vi "AIT 664 - Parse DB.vi"(0 "Path in":path=path "C:/Users/benh/Desktop/Simple Device Export.xml", 11 "error in (no error)":errorcluster) -> (4 "664 Device":T1, 15 "error out":errorcluster)   [LabVIEW 2015, in "AIT 664 Custom Device.lvlib"]
doc: "Read in xml configuration file and merge with params file if it exists"
uses:
  AIT 664 Custom Device.lvlib
  Controls/664 - XML Device Description.ctl
  Controls/664 - XML End System Description.ctl
  Controls/664 - XML Output VL.ctl
  Controls/664 - XML Tx Message Port.ctl
  Controls/664 - Sampling Type.ctl
  Controls/664 -Param.ctl
  Controls/664 - XML Input VL.ctl
  Controls/664 - XML Rx Message Port.ctl
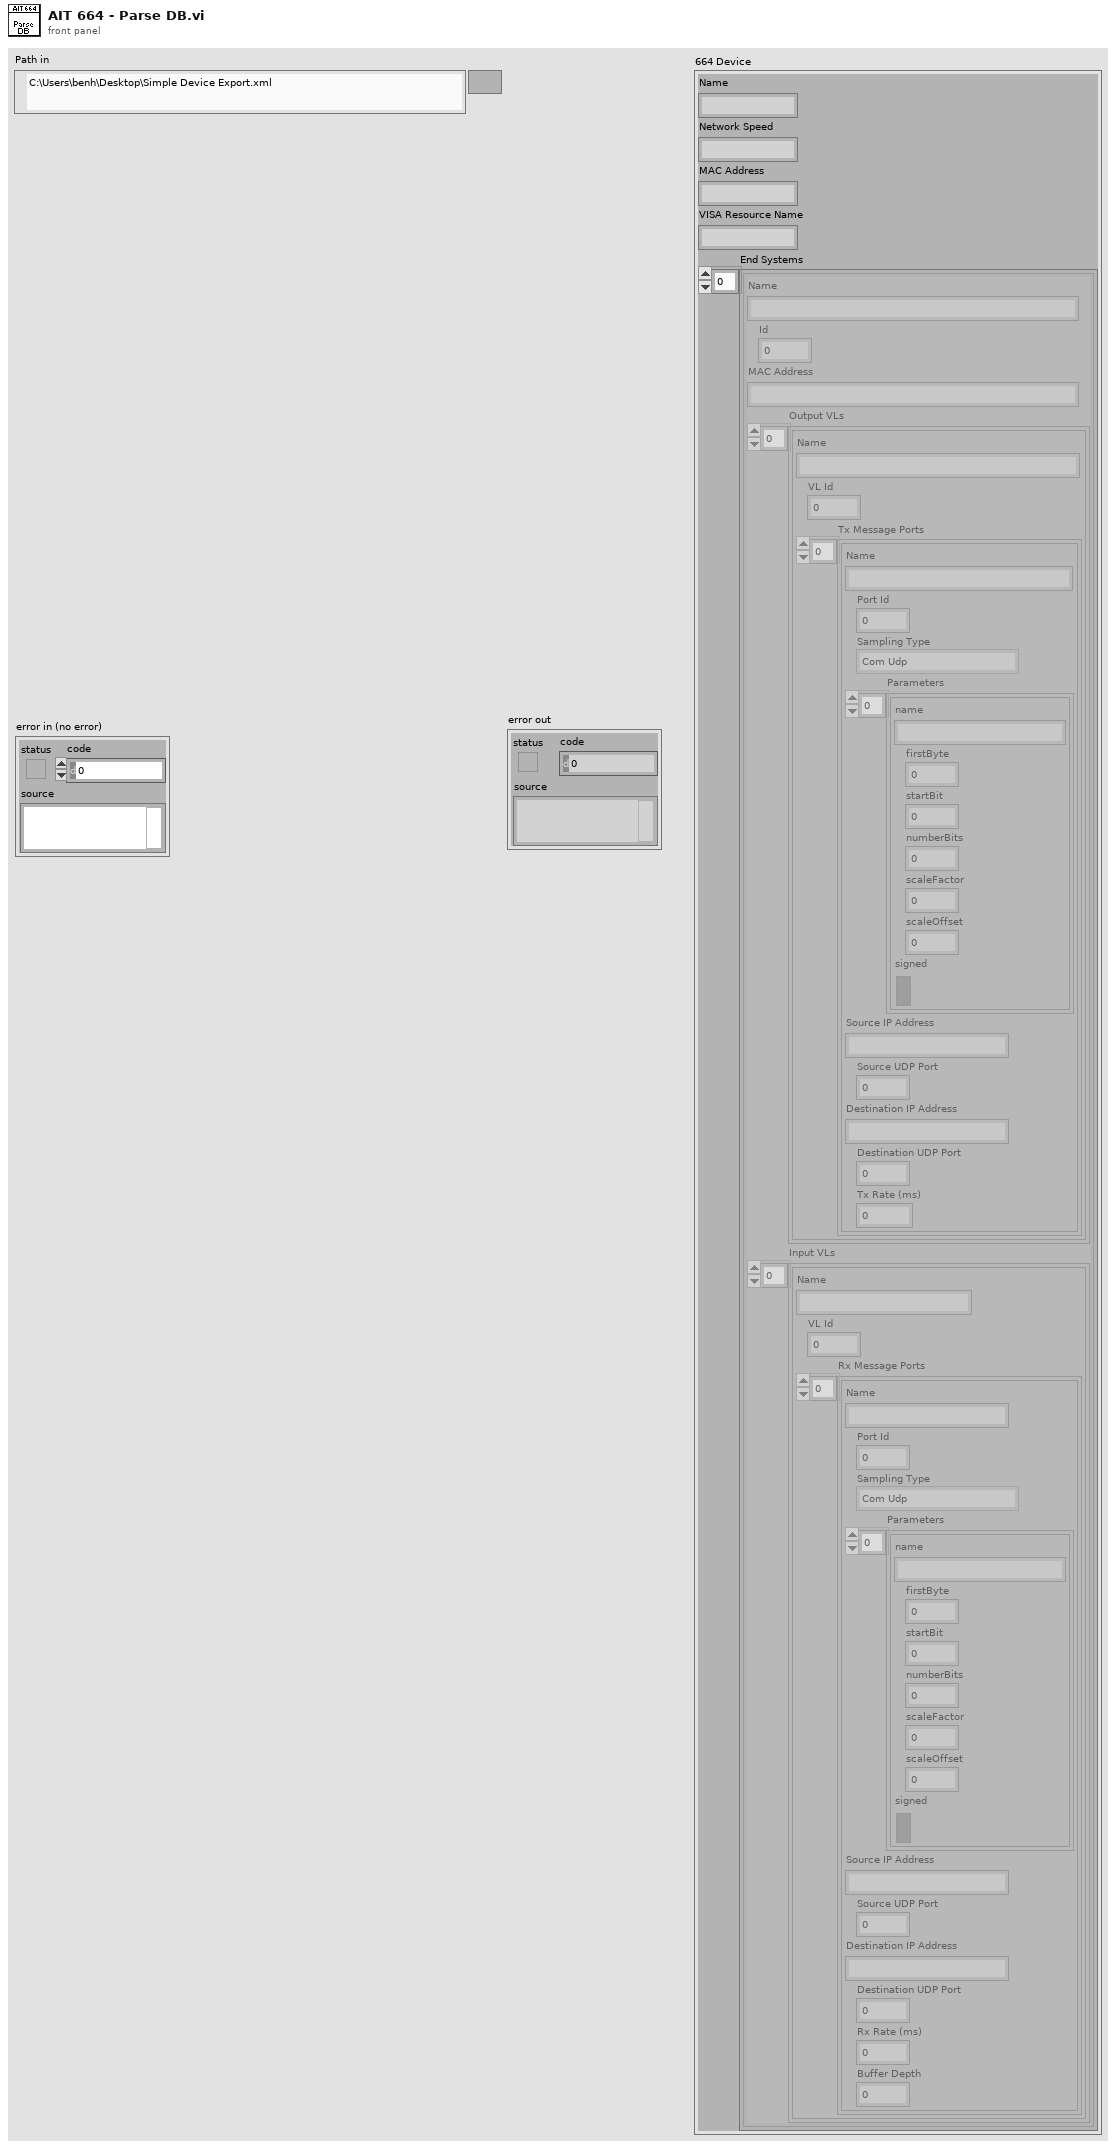
[diagram p1: front panel]
types:
  T1 = typedef "AIT 664 Custom Device.lvlib/664 - XML Device Description.ctl" = cluster{"Name":string, "Network Speed":string, "MAC Address":string, "VISA Resource Name":string, "End Systems":T2[]}
  T2 = typedef "AIT 664 Custom Device.lvlib/664 - XML End System Description.ctl" = cluster{"Name":string, "Id":u32, "MAC Address":string, "Output VLs":T3[], "Input VLs":T7[]}
  T3 = typedef "AIT 664 Custom Device.lvlib/664 - XML Output VL.ctl" = cluster{"Name":string, "VL Id":u32, "Tx Message Ports":T4[]}
  T4 = typedef "AIT 664 Custom Device.lvlib/664 - XML Tx Message Port.ctl" = cluster{"Name":string, "Port Id":u32, "Sampling Type":T5, "Parameters":T6[], "Source IP Address":string, "Source UDP Port":u32, "Destination IP Address":string, "Destination UDP Port":u32, "Tx Rate (ms)":u32}
  T5 = typedef "AIT 664 Custom Device.lvlib/664 - Sampling Type.ctl" = enum16{"Com Udp", "Com Udp Queuing", "Sap Udp", "Sap Ip", "Sap Mac", "Unknown"}
  T6 = typedef "AIT 664 Custom Device.lvlib/664 -Param.ctl" = cluster{"name":string, "firstByte":i32, "startBit":i32, "numberBits":i32, "scaleFactor":dbl, "scaleOffset":dbl, "signed":bool}
  T7 = typedef "AIT 664 Custom Device.lvlib/664 - XML Input VL.ctl" = cluster{"Name":string, "VL Id":u32, "Rx Message Ports":T8[]}
  T8 = typedef "AIT 664 Custom Device.lvlib/664 - XML Rx Message Port.ctl" = cluster{"Name":string, "Port Id":u32, "Sampling Type":T5, "Parameters":T6[], "Source IP Address":string, "Source UDP Port":u32, "Destination IP Address":string, "Destination UDP Port":u32, "Rx Rate (ms)":u32, "Buffer Depth":u32}
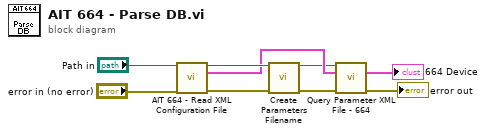
[diagram p0: block diagram]
diagram:
  n1 = call "AIT 664 - Read XML Configuration File.vi"("Path"="Path in", "error in (no error)"="error in (no error)") -> ("Path out"=w7:path, "664 Device"=w4:T1, "error out"=w5:errorcluster)  [unwired: 11 in]
  n2 = call "Create Parameters Filename.vi"("Simulyzer File Path"=w7, "error in (no error)"=w5) -> ("Parm File Path"=w1:path, "error out"=w2:errorcluster)  [unwired: 12 in]
  n3 = call "Query Parameter XML File - 664.vi"("Path in"=w1, "664 Device Without Parameters"=w4, "error in (no error)"=w2) -> ("664 Device With Parameters Out"=→"664 Device":T1, "error out"=→"error out":errorcluster)  [unwired: 11 in]
